vi "AddGroupAndChannelToError.vi"(3 "error in (no error)":errorcluster, 7 "channel name in":string, 9 "group name in":string, 11 "Refnum in":refnum<k34>) -> (17 "error out":errorcluster)   [LabVIEW 2017, in "Tdms.lvlib"]
uses:
  <vilib>/addons/InsightCM/Utilities/Tdms/Tdms.lvlib
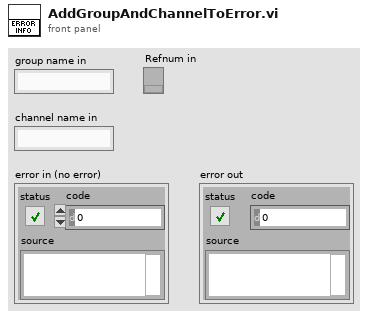
[diagram p1: front panel]
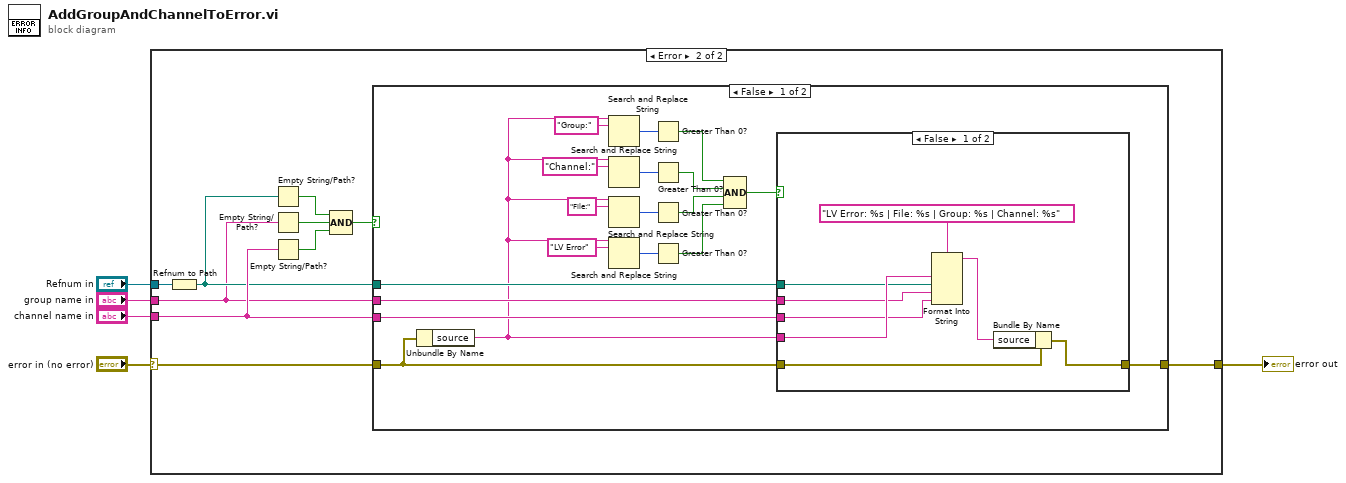
[diagram p0: block diagram]
diagram:
  n1 = case shown="Error" "error in (no error)" {
    selector: "error in (no error)" -> [w6 w15]
    tunnel: "channel name in" -> [_ w13]
    tunnel: "group name in" -> [_ w7]
    tunnel: [w6 w16] -> w3
    tunnel: "Refnum in" -> [_ w14]
    frame No Error {
    }
    frame Error {
      n2 = Refnum to Path(1:w14) -> (0:w8:path)
      n3 = Empty String/Path?(string/path=w8) -> (empty?=w12:bool)
      n4 = Empty String/Path?(string/path=w7) -> (empty?=w11:bool)
      n5 = Empty String/Path?(string/path=w13) -> (empty?=w10:bool)
      n6 = Compound Arithmetic op=AND(w12, w11, w10) -> (w9:bool)
      n7 = case shown="False" w9 {
        tunnel: w13 -> [w35 _]
        tunnel: [w34 w45] -> w16
        tunnel: w15 -> [w33 w45]
        tunnel: w8 -> [w32 _]
        tunnel: w7 -> [w31 _]
        frame False {
          n8 = Unbundle By Name(w33) -> ("source"=w18:string)
          n9 = Search and Replace String(input string=w18, search string="Group:") -> (number of replacements=w25:i32)  [unwired: 6 in, 3 out]
          n10 = Search and Replace String(input string=w18, search string="Channel:") -> (number of replacements=w26:i32)  [unwired: 6 in, 3 out]
          n11 = Search and Replace String(input string=w18, search string="File:") -> (number of replacements=w27:i32)  [unwired: 6 in, 3 out]
          n12 = Search and Replace String(input string=w18, search string="LV Error") -> (number of replacements=w20:i32)  [unwired: 6 in, 3 out]
          n13 = Greater Than 0?(x=w25) -> (x > 0?=w23:bool)
          n14 = Greater Than 0?(x=w26) -> (x > 0?=w24:bool)
          n15 = Greater Than 0?(x=w27) -> (x > 0?=w22:bool)
          n16 = Greater Than 0?(x=w20) -> (x > 0?=w17:bool)
          n17 = Compound Arithmetic op=AND(w23, w24, w22, w17) -> (w21:bool)
          n18 = case shown="False" w21 {
            tunnel: w35 -> [w36 _]
            tunnel: [w42 w44] -> w34
            tunnel: w33 -> [w41 w44]
            tunnel: w32 -> [w38 _]
            tunnel: w31 -> [w37 _]
            tunnel: w18 -> [w39 _]
            frame False {
              n19 = Format Into String(format string="LV Error: %s | File: %s | Group: %s | Channel: %s", w39, w38, w37, w36) -> (resulting string=w40:string)  [unwired: 2 in, 1 out]
              n20 = Bundle By Name(cluster=w41, "source"=w40) -> (w42:errorcluster)
            }
            frame True {
            }
          }
        }
        frame True {
        }
      }
    }
  }
  "error out" <- w3
